vi "RPC Method GreeterService GetFeature.vi"(3 "error in (no error)":errorcluster, 4 "gRPCid in":T1, 5 "DNL_LabVIEW Object in":refnum<class "GreeterServiceImpl.lvclass">) -> (0 "error out":errorcluster, 1 "gRPCid out":T1, 2 "DNL_LabVIEW Object out":refnum<class "GreeterServiceImpl.lvclass">)   [LabVIEW 2019, in "UserCode_impl_server.lvlib" / "GreeterServiceImpl.lvclass"]
uses:
  GreeterServiceImpl.lvclass
  <vilib>/gRPC/LabVIEW gRPC Library/Shared/grpcId.ctl
  Generated_stub_server/RPC Messages/Greeter_res.ctl
  Generated_stub_server/RPC Messages/Greeter_res_res_oneof/Greeter_res_res_oneof.lvclass
  Generated_stub_server/RPC Messages/Greeter_req_req_oneof/Greeter_req_req_oneof.lvclass/Greeter_req_req_oneof.ctl
  Generated_stub_server/RPC Messages/Greeter_MessageA.ctl
  Generated_stub_server/RPC Messages/Greeter_MessageA_oneof_a/Greeter_MessageA_oneof_a.lvclass
  Generated_stub_server/RPC Messages/Greeter_MessageA_oneof_a/Greeter_MessageA_oneof_a.lvclass/Greeter_MessageA_oneof_a.ctl
  Generated_stub_server/RPC Messages/Greeter_res_res_oneof/Greeter_res_res_oneof.lvclass/Greeter_res_res_oneof.ctl
  Generated_stub_server/RPC Service/GreeterServiceStub/GreeterServiceStub.lvclass
  Generated_stub_server/RPC Messages/Greeter_req_req_oneof/Greeter_req_req_oneof.lvclass
  Generated_stub_server/Generated_stub_server.lvlib
  <vilib>/gRPC/LabVIEW gRPC Library/grpc-lvsupport-release.lvlib
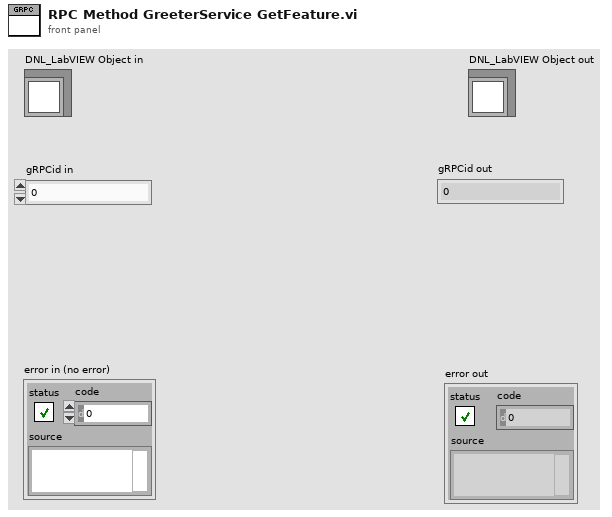
[diagram p1: front panel]
types:
  T1 = typedef "grpc-lvsupport-release.lvlib/grpcId.ctl" = u64
  T2 = typedef "Generated_stub_server.lvlib/Greeter_res.ctl" = cluster{"res_id":i32, "Greeter_res_res_oneof":refnum<class "Greeter_res_res_oneof.lvclass">}
  T3 = typedef "Generated_stub_server.lvlib/Greeter_req.ctl" = cluster{"req_id":i32, "Greeter_req_req_oneof":refnum<class "Greeter_req_req_oneof.lvclass">}
  T4 = typedef "Generated_stub_server.lvlib/Greeter_MessageA.ctl" = cluster{"anotherField":string, "Greeter_MessageA_oneof_a":refnum<class "Greeter_MessageA_oneof_a.lvclass">}
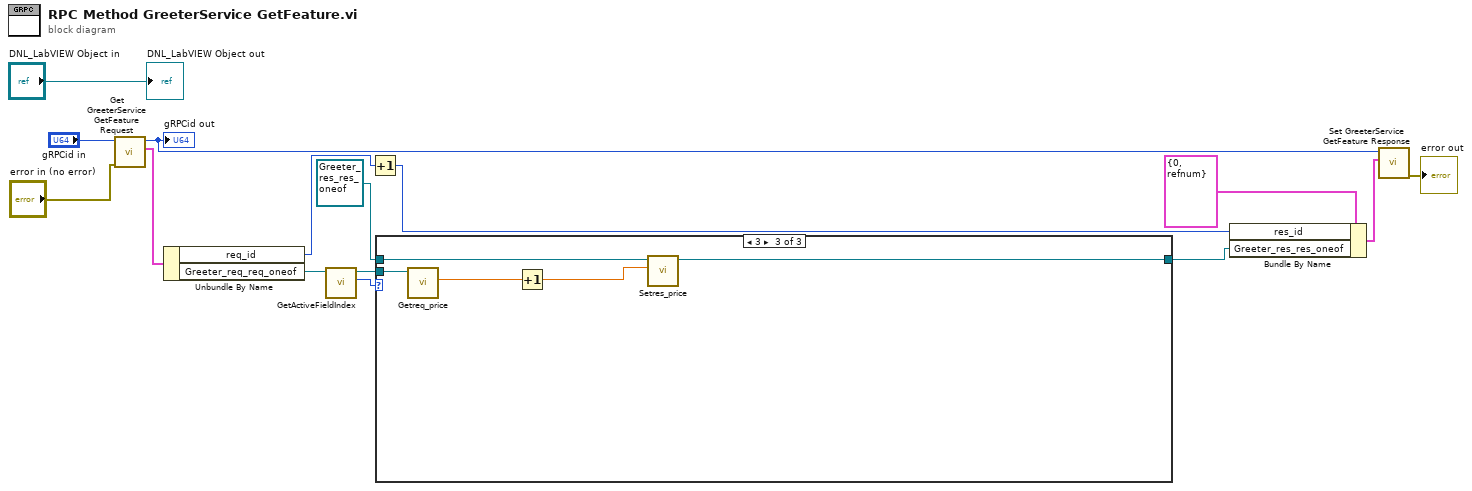
[diagram p0: block diagram]
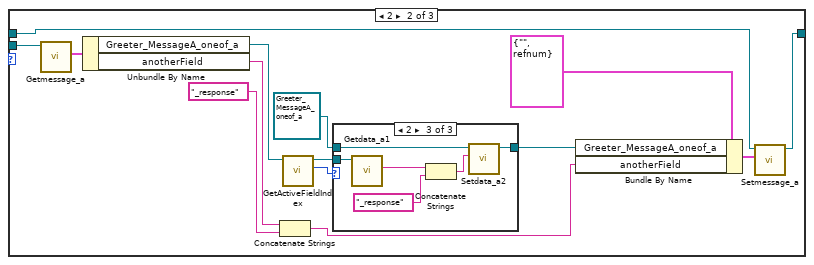
[diagram p3: hidden frame]
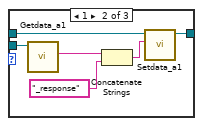
[diagram p5: hidden frame]
diagram:
  n1 = call "Get GreeterService GetFeature Request.vi"("error in (no error)"="error in (no error)", "gRPCid"="gRPCid in") -> ("Message Data"=w15:T3, "gRPCid out"=w4:T1)  [unwired: 7 in, 1 out]
  "gRPCid out" <- w4
  n2 = Unbundle By Name(w15) -> ("req_id"=w10:i32, "Greeter_req_req_oneof"=w13:refnum<class "Greeter_req_req_oneof.lvclass">)
  n3 = call "GetActiveFieldIndex.vi"("OneOfTemplate in"=w13) -> ("Active Field Index"=w11:i32, "OneOfTemplate out"=w12:refnum<class "Greeter_req_req_oneof.lvclass">)  [unwired: 8 in, 1 out]
  n4 = Increment(x=w10) -> (x+1=w6:i32)
  n5 = case shown="3" w11 {
    tunnel: w12 -> [_ w26 w48]
    tunnel: [w16 w25 w44] -> w8
    tunnel: refnum<class "Greeter_res_res_oneof.lvclass"> refnum ("OneOfTemplate in") -> [w16 w24 w45]
    frame 0, Default {
    }
    frame 2 {
      n6 = call "Getmessage_a.vi"("OneOfTemplate in"=w26) -> ("Get_Val"=w30:T4)  [unwired: 8 in, 2 out]
      n7 = Unbundle By Name(w30) -> ("Greeter_MessageA_oneof_a"=w29:refnum<class "Greeter_MessageA_oneof_a.lvclass">, "anotherField"=w19:string)
      n8 = Concatenate Strings(w19, "_response" ("string")) -> (w18:string)
      n9 = call "GetActiveFieldIndex.vi"("OneOfTemplate in"=w29) -> ("Active Field Index"=w28:i32, "OneOfTemplate out"=w27:refnum<class "Greeter_MessageA_oneof_a.lvclass">)  [unwired: 8 in, 1 out]
      n10 = case shown="2" w28 {
        tunnel: w27 -> [_ w37 w42]
        tunnel: refnum<class "Greeter_MessageA_oneof_a.lvclass"> refnum ("OneOfTemplate in") -> [w31 w33 w39]
        tunnel: [w31 w32 w38] -> w22
        frame 0, Default {
        }
        frame 1 {
          n11 = call "Getdata_a1.vi"("OneOfTemplate in"=w37) -> ("Get_Val"=w36:string)  [unwired: 8 in, 2 out]
          n12 = Concatenate Strings(w36, "_response" ("string")) -> (w34:string)
          n13 = call "Setdata_a1.vi"("Set_Val"=w34, "OneOfTemplate in"=w33) -> ("OneOfTemplate out"=w32:refnum<class "Greeter_MessageA_oneof_a.lvclass">)  [unwired: 8 in, 1 out]
        }
        frame 2 {
          n14 = call "Getdata_a1.vi"("OneOfTemplate in"=w42) -> ("Get_Val"=w41:string)  [unwired: 8 in, 2 out]
          n15 = Concatenate Strings(w41, "_response" ("string")) -> (w40:string)
          n16 = call "Setdata_a2.vi"("Set_Val"=w40, "OneOfTemplate in"=w39) -> ("OneOfTemplate out"=w38:refnum<class "Greeter_MessageA_oneof_a.lvclass">)  [unwired: 8 in, 1 out]
        }
      }
      n17 = Bundle By Name(cluster=T4 {"anotherField"="", "Greeter_MessageA_oneof_a"=refnum} ("Greeter_MessageA"), "Greeter_MessageA_oneof_a"=w22, "anotherField"=w18) -> (w20:T4)
      n18 = call "Setmessage_a.vi"("Set_Val"=w20, "OneOfTemplate in"=w24) -> ("OneOfTemplate out"=w25:refnum<class "Greeter_res_res_oneof.lvclass">)  [unwired: 8 in, 1 out]
    }
    frame 3 {
      n19 = call "Getreq_price.vi"("OneOfTemplate in"=w48) -> ("Get_Val"=w47:dbl)  [unwired: 8 in, 2 out]
      n20 = Increment(x=w47) -> (x+1=w46:dbl)
      n21 = call "Setres_price.vi"("Set_Val"=w46, "OneOfTemplate in"=w45) -> ("OneOfTemplate out"=w44:refnum<class "Greeter_res_res_oneof.lvclass">)  [unwired: 8 in, 1 out]
    }
  }
  n22 = Bundle By Name(cluster=T2 {"res_id"=0, "Greeter_res_res_oneof"=refnum} ("Greeter_res"), "res_id"=w6, "Greeter_res_res_oneof"=w8) -> (w9:T2)
  n23 = call "Set GreeterService GetFeature Response.vi"("Message Data"=w9, "gRPCid in"=w4) -> ("error out"=→"error out":errorcluster)  [unwired: 9 in]
  "DNL_LabVIEW Object out" <- "DNL_LabVIEW Object in"
